vi "Get Hierarchy Items.vi"(8 "错误输入（无错误）":errorcluster, 11 "Section in":refnum<data-value>) -> (0 "错误输出":errorcluster, 1 "Names":string[](array[string]), 2 "Items":refnum<data-value>[](array[refnum]), 3 "Section out":refnum<data-value>)   [LabVIEW 2013, in "Hierarchy Framework.lvlib" / "Section.lvclass"]
uses:
  Section.lvclass
  Item/Item.lvclass
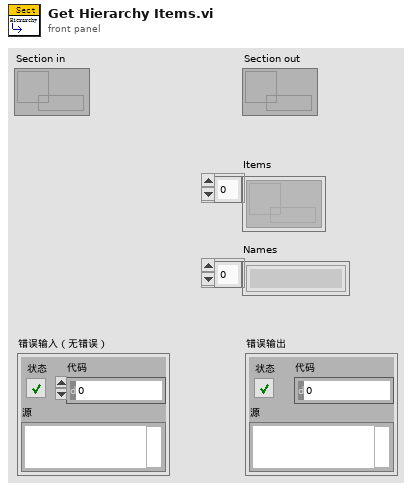
[diagram p1: front panel]
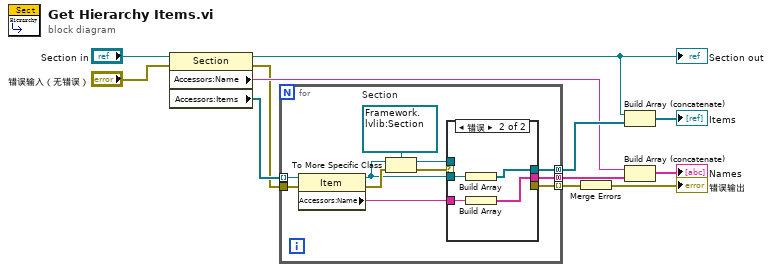
[diagram p0: block diagram]
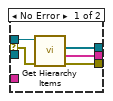
[diagram p2: hidden frame]
diagram:
  n1 = property class="Section"(reference="Section in", error in="错误输入（无错误）") -> (reference out=w9:refnum<data-value>, error out=w3:errorcluster, "Accessors:Name"=w5:string, "Accessors:Items"=w11:refnum<data-value>[])
  "Section out" <- w9
  n2 = for {
    tunnel: w11 -> [w22] mode=indexing
    tunnel: [w16] -> w10 mode=concatenating
    tunnel: [w15] -> w8 mode=concatenating
    tunnel: w3 -> [w14]
    tunnel: [w13] -> w2 mode=indexing
    w23 = refnum<data-value> refnum  # Section
    n3 = property class="Item"(reference=w22, error in=w14) -> (reference out=w17:refnum<data-value>, error out=w21:errorcluster, "Accessors:Name"=w18:string)
    n4 = To More Specific Class(target class=w23, reference=w17, error in=w21) -> (specific class reference=w19:refnum<data-value>, error out=w20:errorcluster)
    n5 = case shown="错误" w20 {
      selector: w20 -> [w27 _]
      tunnel: w19 -> [w28 _]
      tunnel: [w26 w31] -> w16
      tunnel: [w25 w29] -> w15
      tunnel: w18 -> [_ w30]
      tunnel: w17 -> [_ w32]
      tunnel: [w24 _] -> w13
      frame No Error {
        n6 = call "Get Hierarchy Items.vi"("错误输入（无错误）"=w27, "Section in"=w28) -> ("错误输出"=w24:errorcluster, "Names"=w25:string[], "Items"=w26:refnum<data-value>[])  [unwired: 6 in, 1 out]
      }
      frame Error {
        n7 = Build Array(w32) -> (w31:refnum<data-value>[])
        n8 = Build Array(w30) -> (w29:string[])
      }
    }
  }
  n9 = Merge Errors(w2) -> (→"错误输出":errorcluster)
  n10 = Build Array (concatenate)(w9, w10) -> (→"Items":refnum<data-value>[])
  n11 = Build Array (concatenate)(w5, w8) -> (→"Names":string[])
